vi "Read Limit Interval.vi"(8 "error in (no error)":errorcluster, 11 "ACreditAccount in":refnum<class "ACreditAccount.lvclass">) -> (0 "error out":errorcluster, 2 "Limit Interval":u32, 3 "ACreditAccount out":refnum<class "ACreditAccount.lvclass">)   [LabVIEW 2020]
uses:
  ACreditAccount.lvclass
  C:/projects/budget_LabVIEW/Main Codeline/Software/Code/Shared/AInterestAccount/AInterestAccount.lvclass
  C:/projects/budget_LabVIEW/Main Codeline/Software/Code/shared/AAccount/AAccount.lvclass
  C:/projects/budget_LabVIEW/Main Codeline/Software/Code/shared/IInfoable/IInfoable.lvclass
  C:/projects/budget_LabVIEW/Main Codeline/Software/Code/Shared/IInterest/IInterest.lvclass
  C:/projects/budget_LabVIEW/Main Codeline/Software/Code/Shared/ACreditAccount/ACreditAccount.lvclass
  C:/projects/budget_LabVIEW/Main Codeline/Software/Code/Shared/IBorrowable/IBorrowable.lvclass
  C:/projects/budget_LabVIEW/Main Codeline/Software/Code/Shared/IPayable/IPayable.lvclass
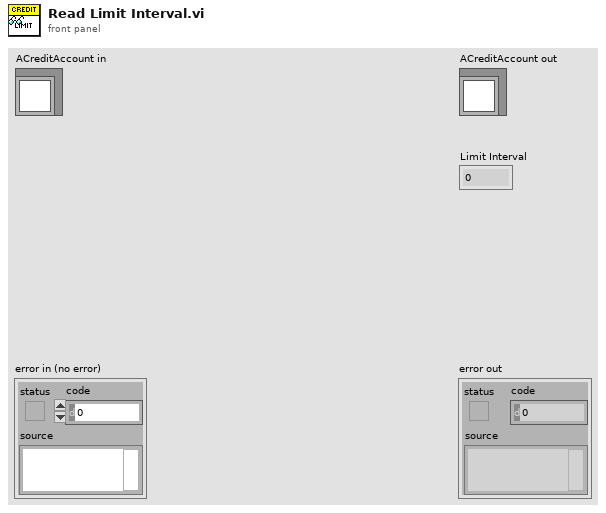
[diagram p1: front panel]
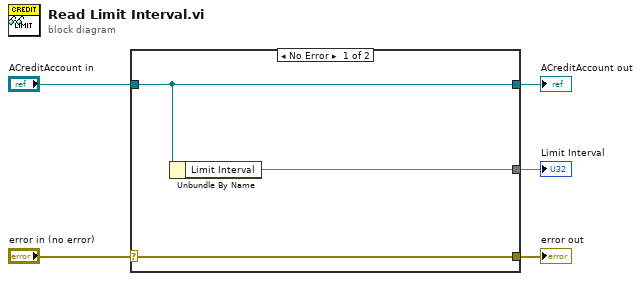
[diagram p0: block diagram]
diagram:
  n1 = case shown="No Error" "error in (no error)" {
    selector: "error in (no error)" -> [w8 w9]
    tunnel: [w8 w9] -> w4
    tunnel: [w7 w10] -> w2
    tunnel: "ACreditAccount in" -> [w7 w10]
    tunnel: [w6 _] -> w1
    frame No Error {
      n2 = Unbundle By Name(w7) -> ("Limit Interval"=w6)
    }
    frame Error {
    }
  }
  "error out" <- w4
  "ACreditAccount out" <- w2
  "Limit Interval" <- w1
